vi "ShipDataJudAndView.vi"(4 "包装箱条码":string, 5 "设定出货数量":string, 6 "箱内产品信息":i32(listbox), 7 "产品种类":enum16{"自产", "外购"}(ring), 8 "error in":errorcluster caption="错误输入", 9 "Debug":bool, 10 "出货数量":refnum<vi>, 11 "箱内产品":refnum<vi>) -> (0 "error out":errorcluster caption="错误输出", 3 "AutoShipFlash":bool)   [LabVIEW 2013]
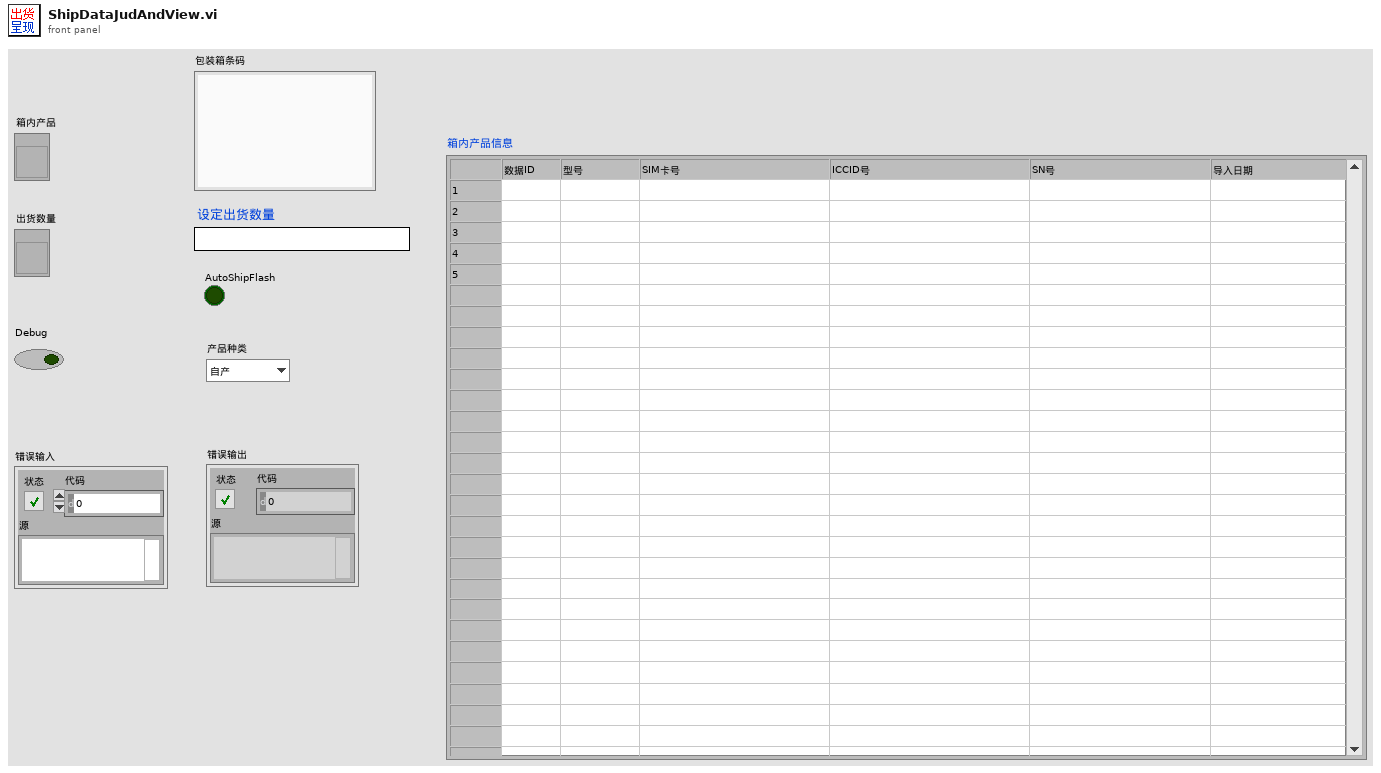
[diagram p1: front panel]
types:
  T1 = typedef "LVRowAndColumnUnsignedTypeDef.ctl" = cluster{"Row":u32, "Column":u32}
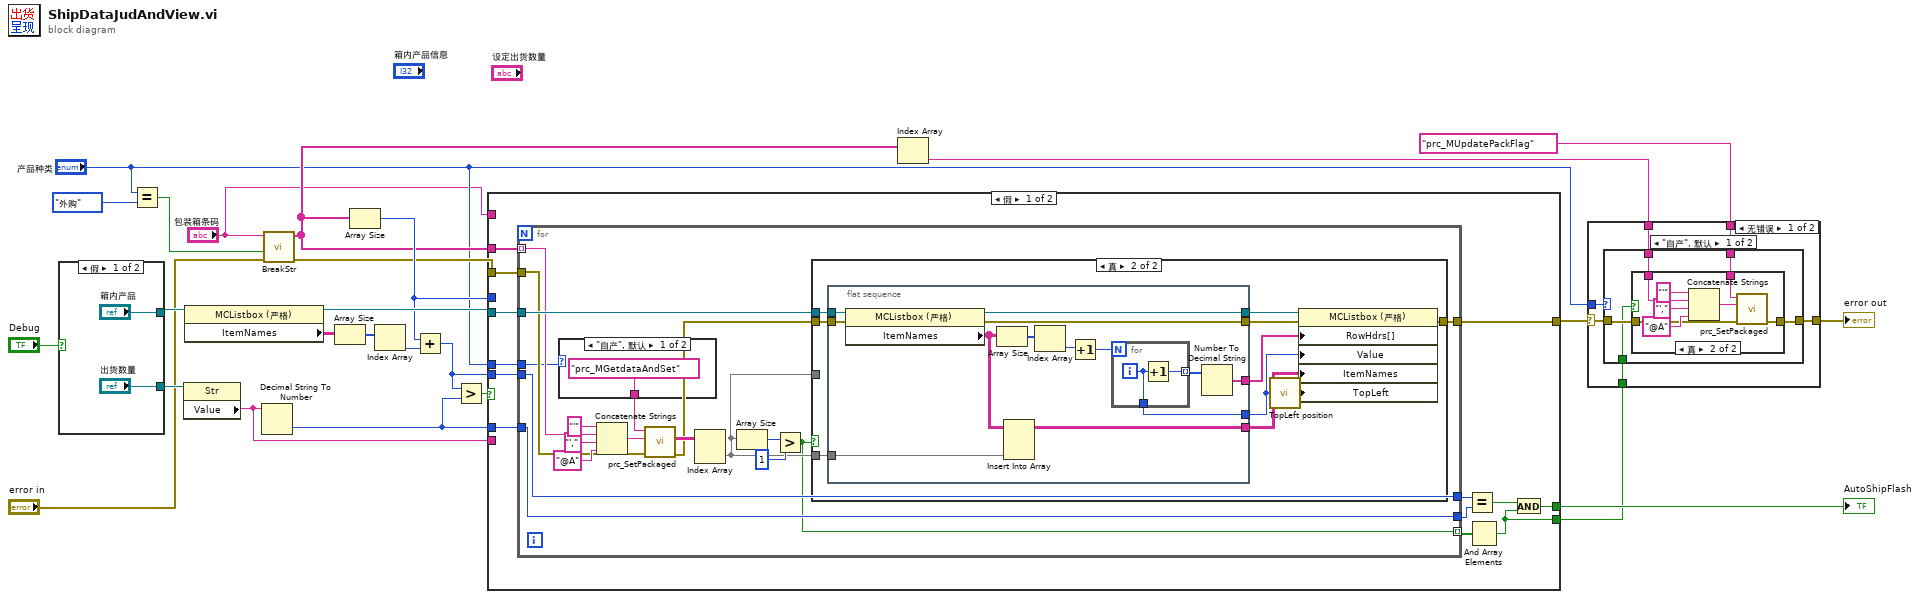
[diagram p0: block diagram]
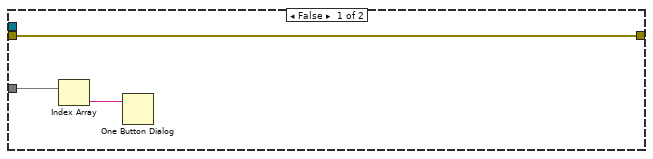
[diagram p5: hidden frame]
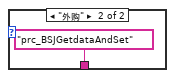
[diagram p6: hidden frame]
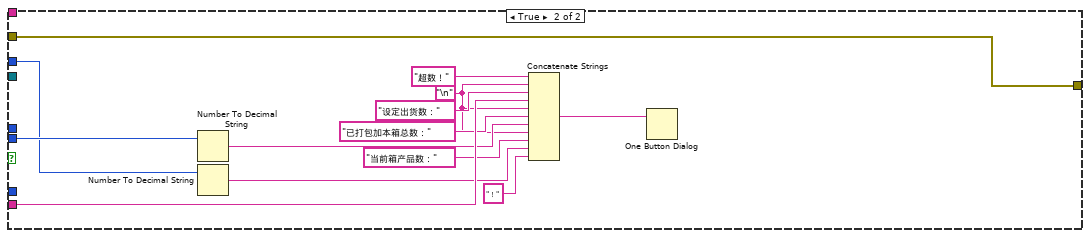
[diagram p7: hidden frame]
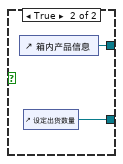
[diagram p8: hidden frame]
diagram:
  n1 = case shown="假" "Debug" {
    tunnel: ["箱内产品" w29] -> w25
    tunnel: ["出货数量" w28] -> w19
    frame False {
    }
    frame True {
      n2 = control-ref of="箱内产品信息"() -> (w29:refnum<vi>)
      n3 = control-ref of="设定出货数量"() -> (w28:refnum<vi>)
    }
  }
  n4 = Equal?(x="产品种类", y=enum16{"自产", "外购"}."外购" ("产品种类")) -> (x = y?=w5:bool)
  n5 = property class="Str"(reference=w19) -> ("Value"=w17:string)  [unwired: 1 in, 2 out]
  n6 = property class="MCListbox (严格)"(reference=w25) -> (reference out=w24:refnum<vi>, "ItemNames"=w23:string[][])  [unwired: 1 in, 1 out]
  n7 = Decimal String To Number(string=w17) -> (number=w4:i32)  [unwired: 2 in, 1 out]
  n8 = call "BreakStr.vi"("error in"="error in", "外购？"=w5, "StrIn"="包装箱条码") -> ("error out"=w14:errorcluster, "ArrayOut"=w11:string[])  [unwired: 7 in]
  n9 = Array Size(array=w23) -> (size(s)=w22:i32[])
  n10 = Array Size(array=w11) -> (size(s)=w16:i32)
  n11 = Index Array(array=w22) -> (element=w21:i32)  [unwired: 1 in]
  n12 = Add(x=w16, y=w21) -> (x+y=w3:i32)
  n13 = Greater?(x=w3, y=w4) -> (0:w18:bool)
  n14 = case shown="假" w18 {
    tunnel: w24 -> [w42 _]
    tunnel: w11 -> [w41 _]
    tunnel: w17 -> [_ w101]
    tunnel: w3 -> [w39 w100]
    tunnel: w16 -> [_ w96]
    tunnel: w14 -> [w40 w91]
    tunnel: w4 -> [w38 _]
    tunnel: [w32 _] -> w13
    tunnel: [w31 w91] -> w8
    tunnel: "产品种类" -> [w35 _]
    tunnel: "包装箱条码" -> [_ _]
    tunnel: [w30 _] -> w1
    frame False {
      n15 = for {
        tunnel: w41 -> [w56] mode=indexing
        tunnel: w42 -> [w58]
        tunnel: w40 -> [w52]
        tunnel: w39 -> [w49]
        tunnel: w38 -> [w48]
        tunnel: [w50] -> w31
        tunnel: [w49] -> w36
        tunnel: [w48] -> w37
        tunnel: w35 -> [w47]
        tunnel: [w43] -> w34 mode=indexing
        n16 = case shown="\"自产\", 默认" w47 {
          tunnel: ["prc_MGetdataAndSet" ("SQL query") "prc_BSJGetdataAndSet" ("SQL query")] -> w60
          frame "自产", Default {
          }
          frame "外购" {
          }
        }
        n17 = Concatenate Strings("'", w56, "',", "@A") -> (w54:string)
        n18 = call "prc_SetPackaged.vi"("error in"=w52, "string"=w54, "SQL query"=w60) -> ("error out"=w51:errorcluster, "Array"=w59:string[][])  [unwired: 7 in]
        n19 = Index Array(array=w59) -> (element=w44:string[])  [unwired: 2 in]
        n20 = Array Size(array=w44) -> (size(s)=w46:i32)
        n21 = Greater?(x=w46, y=1) -> (0:w43:bool)
        n22 = case shown="真" w43 {
          tunnel: w58 -> [_ w67]
          tunnel: w51 -> [w61 w66]
          tunnel: [w61 w65] -> w50
          tunnel: w44 -> [_ w64]
          tunnel: w44 -> [w63 _]
          frame False {
            n23 = Index Array(array=w63) -> (element=w62:string)  [unwired: 1 in]
            n24 = One Button Dialog(message=w62) -> ()  [unwired: 1 in, 1 out]
          }
          frame True {
            n25 = flat-sequence {
              tunnel: [w82] -> w73
              tunnel: [w81] -> w72
              tunnel: [w80] -> w69
              tunnel: [w79] -> w71
              tunnel: [w77] -> w68
              tunnel: w64 -> [w76]
              tunnel: w67 -> [w75]
              tunnel: w66 -> [w74]
              frame #0 {
                n26 = property class="MCListbox (严格)"(reference=w75, error in=w74) -> (reference out=w82:refnum<vi>, error out=w77:errorcluster, "ItemNames"=w84:string[][])
                n27 = Array Size(array=w84) -> (size(s)=w85:i32[])
                n28 = Insert Into Array(array=w84, new element=w76) -> (w79:string[][])  [unwired: 2 in]
                n29 = Index Array(array=w85) -> (element=w86:i32)  [unwired: 1 in]
                n30 = Increment(x=w86) -> (x+1=w78:i32)
                n31 = for {
                  N: w78 -> [_]
                  tunnel: [w87] -> w83 mode=indexing
                  tunnel: [w88] -> w80
                  i -> [w88]
                  n32 = Increment(x=w88) -> (x+1=w87:i32)
                }
                n33 = Number To Decimal String(number=w83) -> (decimal integer string=w81:string[])  [unwired: 1 in]
              }
            }
            n34 = call "TopLeft position.vi"("index"=w69) -> ("TopLeft"=w70:T1)
            n35 = property class="MCListbox (严格)"(reference=w73, error in=w68, "RowHdrs[]"=w72, "Value"=w69, "ItemNames"=w71, "TopLeft"=w70) -> (error out=w65:errorcluster)  [unwired: 1 out]
          }
        }
      }
      n36 = Equal?(x=w36, y=w37) -> (x = y?=w33:bool)
      n37 = And Array Elements(Boolean array=w34) -> (logical AND=w30:bool)
      n38 = And(x=w33, y=w30) -> (x .and. y?=w32:bool)
    }
    frame True {
      w95 = "\n"
      n39 = Number To Decimal String(number=w100) -> (decimal integer string=w98:string)  [unwired: 1 in]
      n40 = Number To Decimal String(number=w96) -> (decimal integer string=w93:string)  [unwired: 1 in]
      n41 = Concatenate Strings("超数！" ("字符串"), w95, "设定出货数：" ("字符串"), w101, w95, "已打包加本箱总数：" ("字符串"), w98, w95, "当前箱产品数：" ("字符串"), w93, "！") -> (w97:string)
      n42 = One Button Dialog(message=w97) -> ()  [unwired: 1 in, 1 out]
    }
  }
  "AutoShipFlash" <- w13
  n43 = Index Array(array=w11) -> (element=w10:string)  [unwired: 1 in]
  n44 = case shown="无错误" w8 {
    selector: w8 -> [w105 w125]
    tunnel: "产品种类" -> [w109 _]
    tunnel: [w108 w125] -> w12
    tunnel: w10 -> [w107 _]
    tunnel: "prc_MUpdatePackFlag" ("SQL query") -> [w106 _]
    tunnel: w1 -> [w104 _]
    frame No Error {
      n45 = case shown="\"自产\", 默认" w109 {
        tunnel: w105 -> [w114 w124]
        tunnel: [w113 w124] -> w108
        tunnel: w107 -> [w112 _]
        tunnel: w106 -> [w111 _]
        tunnel: w104 -> [w110 _]
        frame "自产", Default {
          n46 = case shown="真" w110 {
            tunnel: w114 -> [w115 w119]
            tunnel: [w115 w118] -> w113
            tunnel: w112 -> [_ w117]
            tunnel: w111 -> [_ w116]
            frame False {
            }
            frame True {
              n47 = Concatenate Strings("'", w117, "',", "@A") -> (w121:string)
              n48 = call "prc_SetPackaged.vi"("error in"=w119, "string"=w121, "SQL query"=w116) -> ("error out"=w118:errorcluster)  [unwired: 7 in, 1 out]
            }
          }
        }
        frame "外购" {
        }
      }
    }
    frame Error {
    }
  }
  "error out" <- w12
